vi "VG_DCIRCurrent.vi"() -> ()   [LabVIEW 2020]
panel:
  out "DCIR Current":dbl
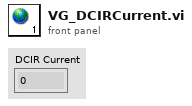
[diagram p1: front panel]
diagram:
